vi "子VI-字符串去除多余0.vi"(11 "带0字符串":string) -> (3 "result string":string caption="去0字符串")   [LabVIEW 2020]
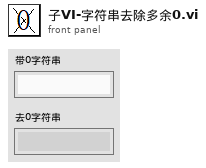
[diagram p1: front panel]
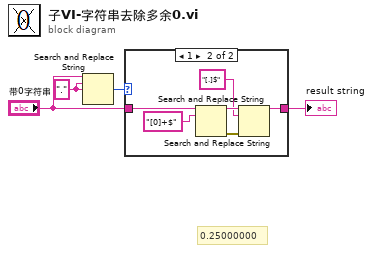
[diagram p0: block diagram]
diagram:
  w4 = "." ("搜索字符串")
  # "0.25000000"
  n1 = Search and Replace String(input string="带0字符串", search string=w4, replace string=w4) -> (number of replacements=w3:i32)  [unwired: 5 in, 3 out]
  n2 = case shown="1" w3 {
    tunnel: "带0字符串" -> [w5 w11]
    tunnel: [w5 w6] -> w1
    frame 0, Default {
    }
    frame 1 {
      n3 = Search and Replace String(input string=w11, search string="[0]+$" ("搜索字符串")) -> (result string=w9:string, error out=w8:errorcluster)  [unwired: 6 in, 2 out]
      n4 = Search and Replace String(input string=w9, search string="[.]$" ("搜索字符串"), error in=w8) -> (result string=w6:string)  [unwired: 5 in, 3 out]
    }
  }
  "result string" <- w1
